vi "Blink test.vi"() -> ()   [LabVIEW 2014]
doc: "Automatically blink and LED attached to a digital output channel of a LINX device."
uses:
  <vilib>/MakerHub/LINX/Public/Peripherals/Digital/Digital Write 1 Chan.vi
  <vilib>/MakerHub/LINX/Public/Peripherals/Digital/Digital Write N Chans.vi
  <vilib>/MakerHub/LINX/Private/Local IO/LinxDigitalWrite.vi
  <vilib>/MakerHub/LINX/Public/Utilities/Check Channel.vi
  <vilib>/MakerHub/LINX/Private/Local IO/Handle Errors.vi
  <vilib>/MakerHub/LINX/Public/Utilities/Open Local.vi
  globals/general globals.vi
  <vilib>/MakerHub/LINX/Private/Utilties/Generate Error.vi
  <vilib>/MakerHub/LINX/LMH-LINX.lvlib
panel:
  out "LED Value":bool
  in  "Digital Output Channel":u8=7
  out "Loop Rate (Hz)":u32
  in  "Stop Button":bool
  # "Circuit Schematic"
  # "LINX Device Settings"
  # "LED Value"
  # "Blink (Serial Interface)\n\nThis example demonstrates how to blink an LED on a LINX device connected to \nthe host computer using USB / Serial.\n\nInstructions\n1. Select the Serial Port associated with the LINX Device.\n2. Select the Digital Pin connected to the LED.\n3. Click the Run Arrow."
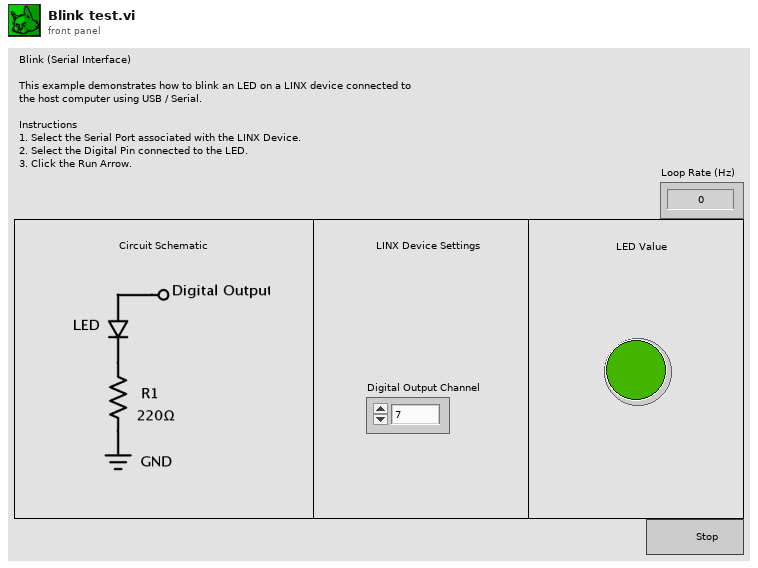
[diagram p1: front panel]
types:
  T1 = typedef "LMH-LINX.lvlib/LINX Ref.ctl" = cluster{"IO":T2, "Interface":T3, "LINX Device Config":T4}
  T2 = typedef "LMH-LINX.lvlib/Platform.ctl" = enum16{"Remote", "Local"}
  T3 = typedef "LMH-LINX.lvlib/Interface.ctl" = enum16{"Serial", "TCP"}
  T4 = typedef "LMH-LINX.lvlib/Device.lvlib/LINX Device Config.ctl" = cluster{"Interface":T3, "COM Port":refnum<visa-resource-name>, "TCP Configuration":T5, "Device Family":u8, "Device ID":u8, "Device Name":string, "TCP Ref":refnum<k5>, "Channels":T6}
  T5 = typedef "LMH-LINX.lvlib/Device.lvlib/TCP Config.ctl" = cluster{"IP Address":string, "Port":u16}
  T6 = typedef "LMH-LINX.lvlib/Channels.ctl" = cluster{"DI":u8[], "DO":u8[], "AI":u8[], "AO":u8[], "PWM":u8[], "QE":u8[], "UART":u8[], "I2C 2":u8[], "SPI":u8[], "CAN":u8[], "Servo":u8[], "AI Ref (V)":dbl, "AI Resolution (Bits)":u8, "AO Ref (V)":dbl, "AO Resolution (Bits)":u8}
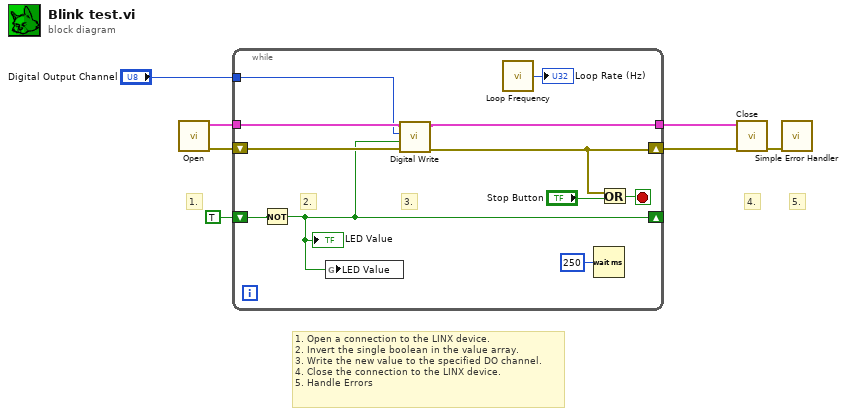
[diagram p0: block diagram]
diagram:
  # "1. Open a connection to the LINX device.\n2. Invert the single boolean in the value array.\n3. Write the new value to the specified DO channel.\n4. Close the connection to the LINX device.\n5. Handle Errors"
  # "5."
  # "4."
  # "1."
  n1 = call-poly <vilib>:"Open.vi"() -> ("Error Out"=w6:errorcluster, "LINX Resource"=w7:T1)  [unwired: 9 in, 1 out]
  n2 = while {
    tunnel: w7 -> [w15]
    tunnel: [w14] -> w5
    shift-right: [w12] -> w4
    shift-left: w6 -> [w13]
    shift-right: [w8] -> _
    shift-left: TRUE -> [w9]
    tunnel: "Digital Output Channel" -> [w10]
    stop <- w18 stop-if-true
    # "2."
    # "3."
    n3 = Not(x=w9) -> (.not. x?=w8:bool)
    "LED Value" <- w8
    n4 = global write "general globals.vi" "LED Value"(w8) -> ()
    n5 = call-poly <vilib>:"Digital Write.vi"("Error In"=w13, "Output Value"=w8, "DO Channel"=w10, "LINX Resource"=w15) -> ("Error Out"=w12:errorcluster, "LINX Resource"=w14:T1)  [unwired: 6 in]
    n6 = call <vilib>:"Loop Frequency.vi"() -> ("Loop Rate (Hz)"=→"Loop Rate (Hz)":u32)
    n7 = Wait (ms)(milliseconds to wait=u32 250) -> ()  [unwired: 1 out]
    n8 = Or(x=w12, y="Stop Button") -> (x .or. y?=w18:bool)
  }
  n9 = call <vilib>:"Close.vi"("Error In"=w4, "LINX Resource"=w5) -> ("Error Out"=w3:errorcluster)  [unwired: 9 in]
  n10 = call <vilib>:"Simple Error Handler.vi"("error in (no error)"=w3) -> ()  [unwired: 4 in, 5 out]
